vi "Install Project.vi"() -> ()   [LabVIEW 2011, in "LVH-Build-Tools.lvlib"]
doc: "This VI will copy the source files into the install directory and create hard links replace the source files with hard links to the install directory.\n\nNote: Do not open any VI's from the source directory. All edits should be done in the Install directory to preserve paths."
uses:
  vi.lib/LabVIEW Hacker/Build Tools/LVH-Build-Tools.lvlib
  vi.lib/LabVIEW Hacker/Build Tools/Private/Type Defs/Install State.ctl
panel:
  out "Tab Control":T1(tab)
  in  "Config Help Button":bool
  in  "Config Settings Button":bool
  in  "Project":u16(ring) items=["lifa", "LIFCK", "LVH-EZ430-Chronos-Interface", "LVH-LINX", "LVH-Toolbox"]
  in  "Configure Cancel":bool
  in  "Configure Next Button":bool
  in  "LabVIEW Version":u16(ring)
  out "Progress Animation":picture
  out "LabVIEW Version":string
  in  "Summary Finish Button":bool
  out "Components Installed":string[](array[string])
  out "Error Out":errorcluster
  # "Install Project\n\nInitializing..."
  # "Install Project\n\nPlease choose a project to install and the version of LabVIEW to install into."
  # "Install Project\n\nInstalling, please wait..."
  # "Install Project\n\nInstallation complete.  Click Finish to exit."
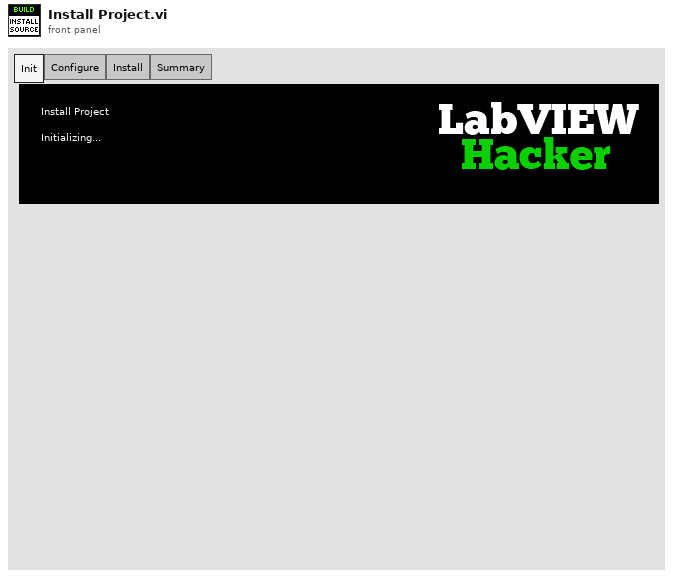
[diagram p1: front panel]
types:
  T1 = enum32{"Init", "Configure", "Install", "Summary"}
  T2 = typedef "LVH-Build-Tools.lvlib/Install State.ctl" = enum16{"Init", "Configure", "Install", "Summary"}
  T3 = typedef "LVH-Build-Tools.lvlib/Sync Source Configuration.ctl" = cluster{"Installed Projects":T4[], "Project Source Root Dir":path, "All Config Files":path[], "Selected Project Config":path, "All LabVIEW Dirs":path[], "Selected LabVIEW Dir":path, "Backup Dir":path}
  T4 = typedef "LVH-Build-Tools.lvlib/Installed Project.ctl" = cluster{"Project Name":string, "LV Versions":T5[], "Project Config Path":path}
  T5 = typedef "LVH-Build-Tools.lvlib/_Installed LabVIEW Version.ctl" = cluster{"Version":string, "Path":path}
  T6 = typedef "LVH-Build-Tools.lvlib/_Animation Config.ctl" = cluster{"Image Data":T7[], "Animation Picture Indicator":refnum<vi>, "FPS":u32, "Position":cluster{"X":i16, "Y":i16}}
  T7 = typedef "imagedata.ctl" = cluster{"image type":i32, "image depth":i32, "image":u8[], "mask":u8[], "colors":u32[], "Rectangle":cluster{"left":i16, "top":i16, "right":i16, "bottom":i16}}
  T8 = typedef "LVH-Build-Tools.lvlib/Configuration.ctl" = cluster{"Source Root":path, "Install Root":string, "Components":string[], "Ignore":string[], "Config Files":path[], "LV Directories":path[], "Install Paths":T9}
  T9 = typedef "LVH-Build-Tools.lvlib/Install Configuration.ctl" = cluster{"LabVIEW Directory":path, "Project Source Config":path}
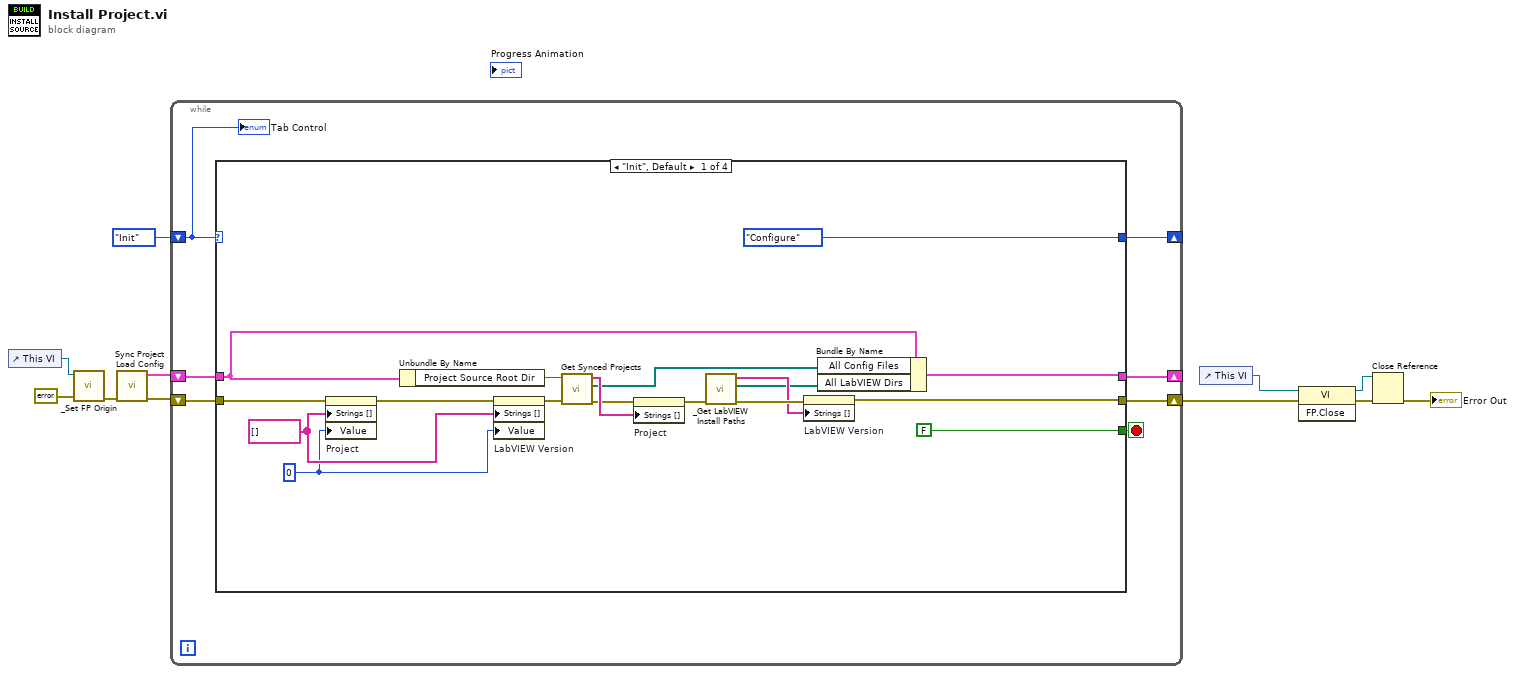
[diagram p0: block diagram]
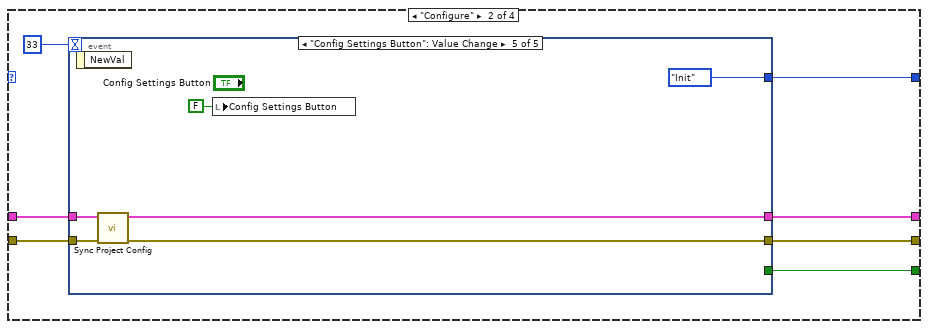
[diagram p2: hidden frame]
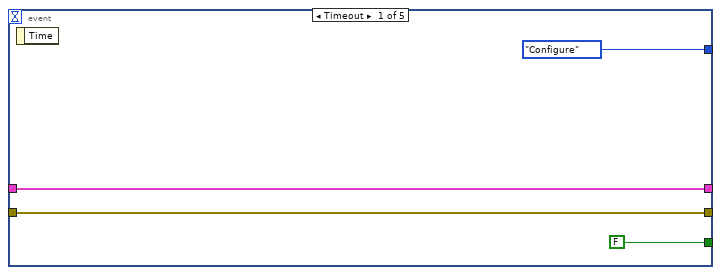
[diagram p3: hidden frame]
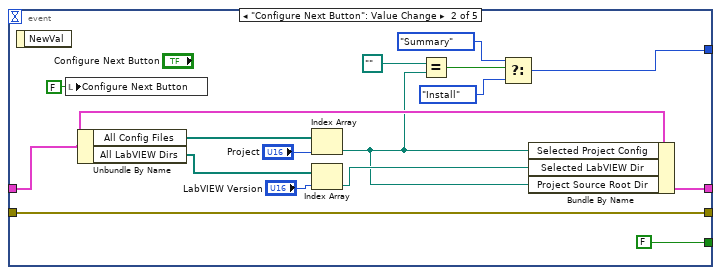
[diagram p4: hidden frame]
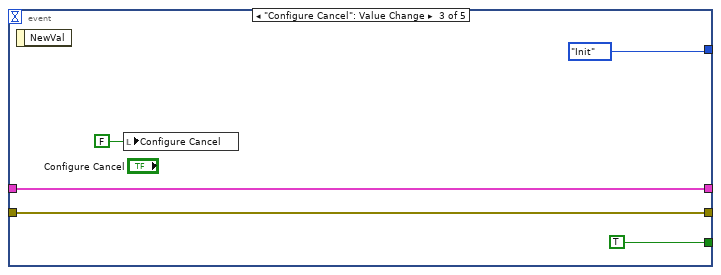
[diagram p5: hidden frame]
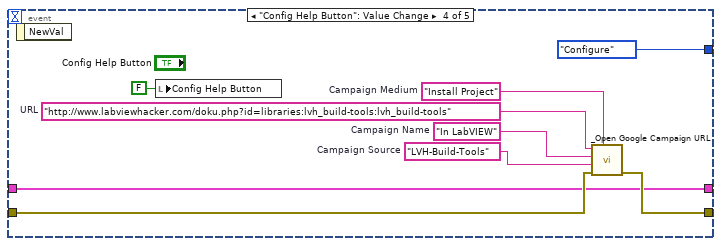
[diagram p6: hidden frame]
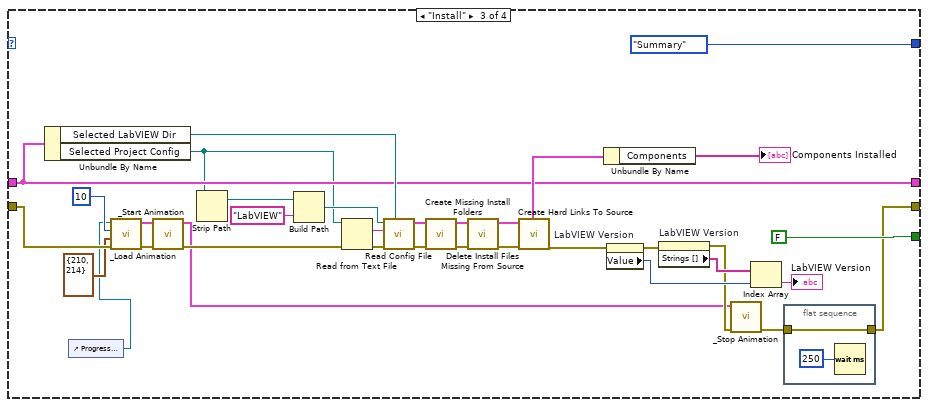
[diagram p7: hidden frame]
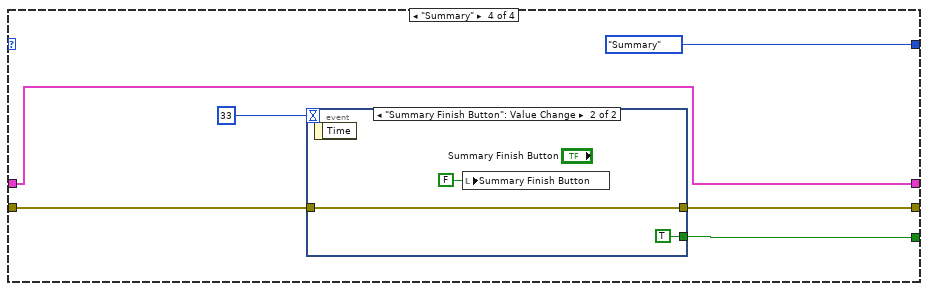
[diagram p8: hidden frame]
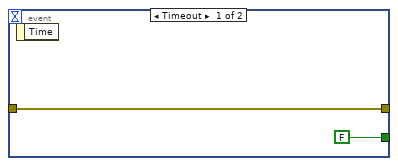
[diagram p9: hidden frame]
diagram:
  n1 = control-ref of="This VI"() -> (w8:refnum<vi>)
  n2 = call "_Set FP Origin.vi"("Error In"=errorcluster {"status"=FALSE, "code"=0, "source"=""} ("Error Out"), "VI Ref"=w8) -> ("Error Out"=w7:errorcluster)  [unwired: 9 in]
  n3 = call "Sync Project Load Config.vi"("Error In"=w7) -> ("Error Out"=w5:errorcluster, "Sync Source Config"=w4:T3)  [unwired: 7 in, 2 out]
  n4 = while {
    shift-right: [w15] -> _
    shift-left: Install_State."Init" ("Install State") -> [w16]
    shift-right: [w17] -> w10
    shift-left: w5 -> [w18]
    shift-right: [w13] -> _
    shift-left: w4 -> [w12]
    stop <- w14 stop-if-true
    n5 = case shown="\"Init\", Default" w16 {
      tunnel: w18 -> [w22 w37 w92 w122]
      tunnel: [w30 w38 w87 w123] -> w17
      tunnel: [Install_State."Configure" ("Install State") w43 Install_State."Summary" ("Install State") Install_State."Summary" ("Install State")] -> w15
      tunnel: [FALSE w41 FALSE w125] -> w14
      tunnel: [w31 w39 w104 w121] -> w13
      tunnel: w12 -> [w25 w40 w104 w121]
      frame "Init", Default {
        w19 = u16 0
        w20 = string[] [] ("Strings []")
        n6 = property on="Project" class="Ring (strict)"(error in=w22, "Strings []"=w20, "Value"=w19) -> (error out=w23:errorcluster)  [unwired: 1 in, 1 out]
        n7 = Unbundle By Name(w25) -> ("Project Source Root Dir"=w24:path)
        n8 = property on="LabVIEW Version" class="Ring (strict)"(error in=w23, "Strings []"=w20, "Value"=w19) -> (error out=w21:errorcluster)  [unwired: 1 in, 1 out]
        n9 = call "Get Synced Projects.vi"("Error In"=w21, "Source Root"=w24) -> ("Error Out"=w32:errorcluster, "Config File Paths"=w29:path[], "Synced Projects"=w34:string[])  [unwired: 7 in]
        n10 = property on="Project" class="Ring (strict)"(error in=w32, "Strings []"=w34) -> (error out=w33:errorcluster)  [unwired: 1 in, 1 out]
        n11 = call "_Get LabVIEW Install Paths.vi"("Error In"=w33) -> ("Error Out"=w36:errorcluster, "LV Directories"=w28:path[], "LV Version"=w35:string[])  [unwired: 8 in]
        n12 = property on="LabVIEW Version" class="Ring (strict)"(error in=w36, "Strings []"=w35) -> (error out=w30:errorcluster)  [unwired: 1 in, 1 out]
        n13 = Bundle By Name(cluster=w25, "All Config Files"=w29, "All LabVIEW Dirs"=w28) -> (w31:T3)
      }
      frame "Configure" {
        n14 = event shown="[4] \"Config Settings Button\": Value Change" {
          selector: _ -> [_ _ _ _ _]
          dyn-events: _ -> [_ _ _ _ _]
          timeout: 33 -> [_ _ _ _ _]
          tunnel: [Install_State."Configure" ("Install State") w49 Install_State."Init" ("Install State") Install_State."Configure" ("Install State") Install_State."Init" ("Install State")] -> w43
          tunnel: [FALSE FALSE TRUE _ _] -> w41
          tunnel: w40 -> [w45 w56 w65 w69 w82]
          tunnel: [w45 w55 w65 w69 w80] -> w39
          tunnel: [w44 w60 w64 w72 w79] -> w38
          tunnel: w37 -> [w44 w60 w64 w71 w81]
          event Timeout {
            n15 = event-data() -> ()  [unwired: 1 in, 1 out]
          }
          event "Configure Next Button": Value Change {
            n16 = event-data() -> ()  [unwired: 1 in, 1 out]
            n17 = local write "Configure Next Button"(FALSE ("Next Button")) -> ()
            n18 = Unbundle By Name(w56) -> ("All Config Files"=w59:path[], "All LabVIEW Dirs"=w58:path[])
            n19 = Index Array(array=w59, index="Project") -> (element=w48:path)
            n20 = Index Array(array=w58, index="LabVIEW Version") -> (element=w57:path)
            n21 = Equal?(x=path "", y=w48) -> (x = y?=w53:bool)
            n22 = Select(t=Install_State."Summary" ("Install State"), s=w53, f=Install_State."Install" ("Install State")) -> (s? t:f=w49:T2)
            n23 = Bundle By Name(cluster=w56, "Selected Project Config"=w48, "Selected LabVIEW Dir"=w57, "Project Source Root Dir"=w48) -> (w55:T3)
          }
          event "Configure Cancel": Value Change {
            n24 = event-data() -> ()  [unwired: 1 in, 1 out]
            n25 = local write "Configure Cancel"(FALSE ("Install Cancel")) -> ()
          }
          event "Config Help Button": Value Change {
            w74 = "LVH-Build-Tools"  # Campaign Source
            w75 = "In LabVIEW"  # Campaign Name
            w76 = "Install Project"  # Campaign Medium
            w70 = "http://www.labviewhacker.com/doku.php?id=libraries:lvh_build-tools:lvh_build-tools"  # URL
            n26 = event-data() -> ()  [unwired: 1 in, 1 out]
            n27 = local write "Config Help Button"(FALSE ("Config Help Button")) -> ()
            n28 = call "_Open Google Campaign URL.vi"("Campaign Medium"=w76, "Error In"=w71, "Campaign Source"=w74, "Campaign Name"=w75, "URL"=w70) -> ("Error Out"=w72:errorcluster)  [unwired: 5 in, 1 out]
          }
          event "Config Settings Button": Value Change {
            n29 = event-data() -> ()  [unwired: 1 in, 1 out]
            n30 = call "Sync Project Config.vi"("Error In"=w81, "Sync Source Config"=w82) -> ("Error Out"=w79:errorcluster, "Sync Source Config"=w80:T3)  [unwired: 8 in]
            n31 = local write "Config Settings Button"(FALSE ("Config Settings Button")) -> ()
          }
        }
      }
      frame "Install" {
        n32 = Unbundle By Name(w104) -> ("Selected LabVIEW Dir"=w107:path, "Selected Project Config"=w95:path)
        n33 = control-ref of="Progress Animation"() -> (w84:refnum<vi>)
        n34 = call "_Load Animation.vi"("Error In"=w92, "Position"=cluster{"X":i16, "Y":i16} {"X"=210, "Y"=214}, "FPS"=u32 10, "Animation Picture Indicator"=w84) -> ("Error Out"=w94:errorcluster, "Animation Config"=w93:T6)  [unwired: 6 in]
        n35 = call "_Start Animation.vi"("Error In"=w94, "Animation Config"=w93) -> ("Error Out"=w89:errorcluster, "Animation Config"=w85:T6)  [unwired: 8 in]
        n36 = Strip Path(path=w95) -> (stripped path=w96:path)  [unwired: 1 out]
        n37 = Build Path(base path=w96, name or relative path="LabVIEW") -> (appended path=w97:path)
        n38 = Read from Text File(file (use dialog)=w95, error in=w89) -> (text=w116:string, error out=w117:errorcluster)  [unwired: 2 in, 2 out]
        n39 = call "Read Config File.vi"("LabVIEW Dir Override"=w107, "error in (no error)"=w117, "Config File In"=w116, "Project Source Root"=w97) -> ("error out"=w115:errorcluster, "Configuration out"=w110:T8)  [unwired: 6 in]
        n40 = call "Create Missing Install Folders.vi"("Error In"=w115, "Configuration"=w110) -> ("Error Out"=w113:errorcluster, "Configuration"=w114:T8)  [unwired: 8 in]
        n41 = call "Delete Install Files Missing From Source.vi"("Error In"=w113, "Configuration"=w114) -> ("Error Out"=w111:errorcluster, "Configuration"=w112:T8)  [unwired: 7 in, 1 out]
        n42 = call "Create Hard Links To Source.vi"("Error In"=w111, "Configuration"=w112) -> ("Error Out"=w101:errorcluster, "Configuration"=w106:T8)  [unwired: 8 in]
        n43 = Unbundle By Name(w106) -> ("Components"=→"Components Installed":string[])
        n44 = property on="LabVIEW Version" class="Ring (strict)"(error in=w101) -> (error out=w100:errorcluster, "Value"=w102:u16)  [unwired: 1 in, 1 out]
        n45 = property on="LabVIEW Version" class="Ring (strict)"(error in=w100) -> (error out=w86:errorcluster, "Strings []"=w103:string[])  [unwired: 1 in, 1 out]
        n46 = call "_Stop Animation.vi"("Error In"=w86, "Animation Config"=w85) -> ("Error Out"=w88:errorcluster)  [unwired: 9 in]
        n47 = Index Array(array=w103, index=w102) -> (element=→"LabVIEW Version":string)
        n48 = flat-sequence {
          tunnel: [w118] -> w87
          tunnel: w88 -> [w118]
          frame #0 {
            n49 = Wait (ms)(milliseconds to wait=u32 250) -> ()  [unwired: 1 out]
          }
        }
      }
      frame "Summary" {
        n50 = event shown="[1] \"Summary Finish Button\": Value Change" {
          selector: _ -> [_ _]
          dyn-events: _ -> [_ _]
          timeout: 33 -> [_ _]
          tunnel: [FALSE TRUE] -> w125
          tunnel: [w127 w128] -> w123
          tunnel: w122 -> [w127 w128]
          event Timeout {
            n51 = event-data() -> ()  [unwired: 1 in, 1 out]
          }
          event "Summary Finish Button": Value Change {
            n52 = event-data() -> ()  [unwired: 1 in, 1 out]
            n53 = local write "Summary Finish Button"(FALSE ("Summary Finish Button")) -> ()
          }
        }
      }
    }
    "Tab Control" <- w16
  }
  n54 = control-ref of="This VI"() -> (w3:refnum<vi>)
  n55 = invoke class="VI" method="FP.Close"(reference=w3, error in=w10) -> (reference out=w2:refnum<vi>, error out=w1:errorcluster)  [unwired: 1 in, 1 out]
  n56 = Close Reference(reference=w2, error in (no error)=w1) -> (error out=→"Error Out":errorcluster)
